vi "HFRR ADV v08 new software.vi"() -> ()   [LabVIEW 2025] (continued)
          n1265 = Read from Text File "Read File"(file (use dialog)=w1584) -> (text=w1583:string)  [unwired: 3 in, 3 out]
          n1266 = Match Pattern(string=w1583, regular expression="]") -> (after substring=w1581:string)  [unwired: 1 in, 3 out]
          n1267 = String Subset(string=w1583, offset (0)=5, length (rest)=10 ("length (rest)")) -> (substring=w1576:string)
          n1268 = Fract/Exp String To Number(string=w1576) -> (number=w1577:dbl)  [unwired: 3 in, 1 out]
          n1269 = Match Pattern(string=w1581, regular expression="-") -> (before substring=w1579:string)  [unwired: 1 in, 3 out]
          n1270 = case shown="19" w1578 {
            tunnel: w1577 -> [w1587 w1588 w1589 w1590 _ _ _ w1595 w1596 _ w1597 w1598 w1599 w1600 w1601 w1602 _ w1603 w1604 _ _ _ _ _]
            tunnel: w1579 -> [_ _ _ _ w1591 w1592 w1593 _ _ _ _ _ _ _ _ _ _ _ _ w1605 w1606 w1607 w1608 _]
            frame 0 {
              n1271 = local write "FRIC. FORCE :"(w1587) -> ()
            }
            frame 1 {
              n1272 = local write "TEMPERATURE :"(w1588) -> ()
            }
            frame 2 {
              n1273 = local write "HUMIDITY:"(w1589) -> ()
            }
            frame 3 {
              n1274 = local write "AIR TEMPERATURE :"(w1590) -> ()
            }
            frame 4 {
              n1275 = local write "Com Port 1"(w1591) -> ()
            }
            frame 5 {
              n1276 = local write "Com Port 2"(w1592) -> ()
              n1277 = local write "visa due"(w1592) -> ()
            }
            frame 6 {
              n1278 = String To Path(string=w1593) -> (path=w1594:path)
              n1279 = local write "File Path"(w1594) -> ()
              "String" <- w1593
            }
            frame 7 {
              n1280 = local write "DISPLACEMENT :"(w1595) -> ()
            }
            frame 8 {
              n1281 = local write "STROKE GAIN :"(w1596) -> ()
            }
            frame 9 {
            }
            frame 10 {
              n1282 = local write "Language Selection"(w1597) -> ()
            }
            frame 11 {
              n1283 = local write "CH-POWER +"(w1598) -> ()
            }
            frame 12 {
              n1284 = local write "CH-POWER -"(w1599) -> ()
            }
            frame 13 {
              n1285 = local write "CH-HEATER"(w1600) -> ()
            }
            frame 14 {
              n1286 = local write "CH-HUMIDITY WET"(w1601) -> ()
            }
            frame 15 {
              n1287 = local write "CH-HUMIDITY DRY"(w1602) -> ()
            }
            frame 16 {
            }
            frame 17 {
              n1288 = local write "AIR TEMP INTERCEPT:"(w1603) -> ()
            }
            frame 18 {
              n1289 = local write "TEMP INTERCEPT:"(w1604) -> ()
            }
            frame 21 {
              n1290 = local write "S.NO"(w1605) -> ()
            }
            frame 22 {
              n1291 = local write "Com Port 3"(w1606) -> ()
            }
            frame 20 {
              n1292 = local write "Camera Port :"(w1607) -> ()
            }
            frame 19 {
              n1293 = local write "C3 :"(w1608) -> ()
            }
            frame 23, Default {
            }
          }
        }
      }
    }
    n1294 = Select(t=u32 2500 ("milliseconds to wait"), s=w1561, f=u32 500 ("milliseconds to wait")) -> (s? t:f=w1559:u32)
    n1295 = Multiply(x=w1564, y=w1559) -> (x*y=w1566:dbl)
    n1296 = property on="Time slide" class="Slide (strict)"("Visible"=w1555) -> ()  [unwired: 2 in, 2 out]
    n1297 = call "Elapsed Time2"("Time Target (s)"=w1566, "Auto Reset"=TRUE) -> ("Time has Elapsed"=w1556:bool)  [unwired: 10 in, 7 out]
    n1298 = case shown="True" w1556 {
      frame False {
      }
      frame True {
        n1299 = stacked-sequence {
          frame #0 {
            # "DATA PROCESSING"
            # "115 mV/N"
            n1300 = local read "Sample Temperature"() -> (w1609:dbl)
            "TEMP 2" <- w1609
            "TEMP 3" <- w1609
            n1301 = local read "RH Numeric:"() -> (w1616:dbl)
            n1302 = local read "HUMIDITY:"() -> (w1617:dbl)
            n1303 = local read "FRICVALZ"() -> (w1628:dbl)
            n1304 = local read "Friction"() -> (w1612:dbl)
            n1305 = local write "TEMP"(w1609) -> ()
            n1306 = Multiply(x=w1616, y=w1617) -> (x*y=→"Humidity ( %RH )" →"Hum" →"Hum 2":dbl)
            n1307 = Subtract(x=w1612, y=w1628) -> (x-y=w1623:dbl)
            "FF 2" <- w1623
            "FF 4" <- w1623
            n1308 = local read "Ambient Temperature"() -> (→"AIR TEMP":dbl)
            n1309 = local read "TEMP"() -> (w1627:dbl)
            n1310 = local write "FF 3"(w1623) -> ()
            n1311 = Compound Arithmetic op=OR("FRICVALZ 4", "FRICVALZ 3", "FRICVALZ 2") -> (w1619:bool)
            n1312 = case shown="True" w1619 {
              tunnel: w1612 -> [_ w1634]
              frame False {
              }
              frame True {
                w1633 = FALSE ("FRICVALZ")
                n1313 = local write "FRICVALZ 3"(w1633) -> ()
                n1314 = local write "FRICVALZ 2"(w1633) -> ()
                n1315 = local write "FRICVALZ 4"(w1633) -> ()
                "FRICVALZ" <- w1634
              }
            }
            n1316 = Not A Number/Path/Refnum?(number/path/refnum=w1627) -> (NaN/Path/Refnum?=w1626:bool)
            n1317 = Not A Number/Path/Refnum?(number/path/refnum=w1623) -> (NaN/Path/Refnum?=w1625:bool)
            n1318 = Divide(x=w1623, y=1.96) -> (x/y=w1620:dbl)
            n1319 = Compound Arithmetic op=OR(w1626, w1625) -> (w1624:bool)
            n1320 = Not A Number/Path/Refnum?(number/path/refnum=w1620) -> (NaN/Path/Refnum?=w1621:bool)
            n1321 = case shown="True" w1624 {
              frame False {
              }
              frame True {
                n1322 = local write "TEMP"(0.0 ("TEMP")) -> ()
                n1323 = local write "FF 2"(0.0 ("FF 2")) -> ()
                n1324 = local write "reinit"(TRUE ("reinit")) -> ()
              }
            }
            n1325 = Select(t=0.0, s=w1621, f=w1620) -> (s? t:f=w1611:dbl)
            "COF 2" <- w1611
            n1326 = local write "COF 3"(w1611) -> ()
          }
        }
      }
    }
    n1327 = Wait (ms)(milliseconds to wait=u32 50) -> ()  [unwired: 1 out]
    n1328 = local read "Quit"() -> (w1548:bool)
    "Rate" <- 2500.0 ("No of Samples")
  }
  n1329 = while {
    tunnel: w57 -> [_]
    tunnel: [w1661] -> _
    tunnel: [w1637] -> w56
    i -> [w1661]
    stop <- w1637 stop-if-true
    # "C:\\LAB-IQ-NXT\\Scar View.exe"
    n1330 = local read "OK Button 16"() -> (w1650:bool)
    n1331 = local read "Main Tab"() -> (w1643:T2)
    n1332 = local read "service 3"() -> (w1644:bool)
    n1333 = local read "OPEN 6"() -> (w1646:bool)
    n1334 = local read "EDIT 2"() -> (w1648:bool)
    n1335 = flat-sequence {
      frame #0 {
        n1336 = local read "SAVE 2"() -> (w2263:bool)
        n1337 = stacked-sequence {
          frame #0 {
            n1338 = local read "EDIT"() -> (w2317:bool)
            n1339 = case shown="True" w2317 {
              tunnel: [u8 2 ("Disabled") u8 0 ("Disabled")] -> _
              frame False {
                w2319 = FALSE
                n1340 = local write "Password"("") -> ()
                n1341 = property on="SrvM CP" class="Bool (strict)"("Visible"=w2319) -> ()  [unwired: 2 in, 2 out]
                n1342 = property on="message" class="Str"("Visible"=w2319) -> ()  [unwired: 2 in, 2 out]
                n1343 = local write "x = y?"(w2319) -> ()
                n1344 = property on="Password" class="Str"("Visible"=w2319) -> ()  [unwired: 2 in, 2 out]
                n1345 = property on="ENTER THE NEW PASSWORD" class="Str"("Visible"=w2319) -> ()  [unwired: 2 in, 2 out]
                n1346 = property on="ENTER CURRENT PASSWORD" class="Str"("Visible"=w2319) -> ()  [unwired: 2 in, 2 out]
                n1347 = local write "SrvM CP"(w2319) -> ()
              }
              frame True {
                w2322 = TRUE
                n1348 = property on="SrvM CP" class="Bool (strict)"("Visible"=w2322) -> ()  [unwired: 2 in, 2 out]
                n1349 = property on="Password" class="Str"("Visible"=w2322) -> ()  [unwired: 2 in, 2 out]
              }
            }
            "dipl pwd" <- "@143$\n" ("dipl pwd")
          }
          frame #1 {
            # "Gain password"
            n1350 = String To Byte Array(string="ENTER CURRENT PASSWORD") -> (unsigned byte array=w2327:u8[])
            n1351 = Search 1D Array(1D array=w2327, element=u8 10) -> (index of element=w2330:i32)  [unwired: 1 in]
            n1352 = Index Array(array=w2327, index=w2330) -> (element=w2326:u8)
            n1353 = Equal?(x=w2326, y=10) -> (x = y?=w2324:bool)
            n1354 = case shown="True" w2324 {
              frame False {
                n1355 = property on="ENTER THE NEW PASSWORD" class="Str"("Visible"=FALSE) -> ()  [unwired: 2 in, 2 out]
              }
              frame True {
                # "password"
                # "change password logic"
                n1356 = local read "ENTER CURRENT PASSWORD"() -> (w2343:string)
                n1357 = local read "dipl pwd"() -> (w2337:string)
                n1358 = String To Byte Array(string=w2343) -> (unsigned byte array=w2345:u8[])
                n1359 = String To Byte Array(string=w2337) -> (unsigned byte array=w2338:u8[])
                n1360 = Array Size(array=w2345) -> (size(s)=w2342:i32)
                n1361 = Array Size(array=w2338) -> (size(s)=w2340:i32)
                n1362 = for {
                  N: w2342 -> [_]
                  tunnel: w2345 -> [w2369]
                  tunnel: [w2367] -> w2346 mode=indexing
                  tunnel: w2342 -> [w2361]
                  i -> [w2362]
                  n1363 = Decrement(x=w2361) -> (x-1=w2359:i32)
                  n1364 = Equal?(x=w2362, y=w2359) -> (x = y?=w2360:bool)
                  n1365 = Index Array(array=w2369, index=w2362) -> (element=w2363:u8)
                  n1366 = Number To Decimal String(number=w2363) -> (decimal integer string=w2368:string)  [unwired: 1 in]
                  n1367 = Select(t="", s=w2360, f="\r") -> (s? t:f=w2365:string)
                  n1368 = Concatenate Strings(w2368, w2365) -> (w2367:string)
                }
                n1369 = for {
                  N: w2340 -> [_]
                  tunnel: w2338 -> [w2357]
                  tunnel: [w2355] -> w2339 mode=indexing
                  tunnel: w2340 -> [w2352]
                  i -> [w2353]
                  n1370 = Decrement(x=w2352) -> (x-1=w2351:i32)
                  n1371 = Equal?(x=w2353, y=w2351) -> (x = y?=w2350:bool)
                  n1372 = Index Array(array=w2357, index=w2353) -> (element=w2356:u8)
                  n1373 = Number To Decimal String(number=w2356) -> (decimal integer string=w2354:string)  [unwired: 1 in]
                  n1374 = Select(t="", s=w2350, f="\r") -> (s? t:f=w2347:string)
                  n1375 = Concatenate Strings(w2354, w2347) -> (w2355:string)
                }
                n1376 = local read "string"() -> (w2344:string)
                n1377 = Concatenate Strings(w2339) -> (w2333:string)
                n1378 = Concatenate Strings(w2344) -> (w2341:string)
                n1379 = Concatenate Strings(w2346) -> (w2334:string)
                n1380 = Equal?(x=w2334, y=w2341) -> (x = y?=w2336:bool)
                n1381 = Equal?(x=w2334, y=w2333) -> (x = y?=w2332:bool)
                n1382 = Or(x=w2336, y=w2332) -> (x .or. y?=w2335:bool)
                n1383 = case shown="True" w2335 {
                  frame False {
                  }
                  frame True {
                    n1384 = property on="ENTER THE NEW PASSWORD" class="Str"("Visible"=TRUE) -> ()  [unwired: 2 in, 2 out]
                  }
                }
              }
            }
          }
          frame #2 {
            n1385 = String To Byte Array(string="ENTER THE NEW PASSWORD") -> (unsigned byte array=w2372:u8[])
            n1386 = Search 1D Array(1D array=w2372, element=u8 10) -> (index of element=w2376:i32)  [unwired: 1 in]
            n1387 = Index Array(array=w2372, index=w2376) -> (element=w2374:u8)
            n1388 = Equal?(x=w2374, y=10) -> (x = y?=w2371:bool)
            n1389 = case shown="False" w2371 {
              frame False {
              }
              frame True {
                n1390 = local write "EDIT"(FALSE) -> ()
                n1391 = local write "SrvM CP"(FALSE) -> ()
                n1392 = local read "ENTER THE NEW PASSWORD"() -> (w2379:string)
                n1393 = String To Byte Array(string=w2379) -> (unsigned byte array=w2384:u8[])
                n1394 = Array Size(array=w2384) -> (size(s)=w2381:i32)
                n1395 = for {
                  N: w2381 -> [_]
                  tunnel: w2384 -> [w2397]
                  tunnel: [w2394] -> w2386 mode=indexing
                  tunnel: w2381 -> [w2389]
                  i -> [w2387]
                  n1396 = Decrement(x=w2389) -> (x-1=w2390:i32)
                  n1397 = Equal?(x=w2387, y=w2390) -> (x = y?=w2391:bool)
                  n1398 = Index Array(array=w2397, index=w2387) -> (element=w2396:u8)
                  n1399 = Number To Decimal String(number=w2396) -> (decimal integer string=w2395:string)  [unwired: 1 in]
                  n1400 = Select(t="", s=w2391, f="\r") -> (s? t:f=w2388:string)
                  n1401 = Concatenate Strings(w2395, w2388) -> (w2394:string)
                }
                n1402 = local read "file path"() -> (w2378:path)
                n1403 = Concatenate Strings(w2386) -> (w2380:string)
                n1404 = Delete(path (use dialog)=w2378) -> (deleted path=w2382:path)  [unwired: 4 in, 2 out]
                n1405 = call <vilib>:"Write Characters To File.vi"("append to file? (new file:F)"=FALSE, "character string"=w2380, "file path (dialog if empty)"=w2382) -> ()  [unwired: 2 in, 1 out]
              }
            }
          }
          frame #3 {
            n1406 = case shown="True" "SrvM CP" {
              frame False {
                w2400 = ""
                n1407 = local write "ENTER CURRENT PASSWORD"(w2400) -> ()
                n1408 = local write "ENTER THE NEW PASSWORD"(w2400) -> ()
                n1409 = property on="ENTER CURRENT PASSWORD" class="Str"("Visible"=FALSE) -> ()  [unwired: 2 in, 2 out]
              }
              frame True {
                n1410 = property on="ENTER THE NEW PASSWORD" class="Str"() -> ("Visible"=w2401:bool)  [unwired: 2 in, 2 out]
                n1411 = Not(x=w2401) -> (.not. x?=w2402:bool)
                n1412 = property on="ENTER CURRENT PASSWORD" class="Str"("Visible"=w2402) -> ()  [unwired: 2 in, 2 out]
              }
            }
          }
          frame #4 {
            n1413 = String To Byte Array(string="Password") -> (unsigned byte array=w2409:u8[])
            n1414 = Search 1D Array(1D array=w2409, element=u8 10) -> (index of element=w2407:i32)  [unwired: 1 in]
            n1415 = Index Array(array=w2409, index=w2407) -> (element=w2408:u8)
            n1416 = Equal?(x=w2408, y=10) -> (x = y?=w2404:bool)
            n1417 = case shown="True" w2404 {
              frame False {
              }
              frame True {
                # "password"
                # "password"
                n1418 = local read "Password"() -> (w2422:string)
                n1419 = String To Byte Array(string=w2422) -> (unsigned byte array=w2425:u8[])
                n1420 = String To Byte Array(string="@143$\n") -> (unsigned byte array=w2411:u8[])
                n1421 = Array Size(array=w2425) -> (size(s)=w2420:i32)
                n1422 = Array Size(array=w2411) -> (size(s)=w2416:i32)
                n1423 = for {
                  N: w2420 -> [_]
                  tunnel: w2425 -> [w2459]
                  tunnel: [w2457] -> w2426 mode=indexing
                  tunnel: w2420 -> [w2454]
                  i -> [w2455]
                  n1424 = Decrement(x=w2454) -> (x-1=w2453:i32)
                  n1425 = Index Array(array=w2459, index=w2455) -> (element=w2458:u8)
                  n1426 = Equal?(x=w2455, y=w2453) -> (x = y?=w2452:bool)
                  n1427 = Number To Decimal String(number=w2458) -> (decimal integer string=w2456:string)  [unwired: 1 in]
                  n1428 = Select(t="", s=w2452, f="\r") -> (s? t:f=w2449:string)
                  n1429 = Concatenate Strings(w2456, w2449) -> (w2457:string)
                }
                n1430 = for {
                  N: w2416 -> [_]
                  tunnel: w2411 -> [w2470]
                  tunnel: [w2468] -> w2414 mode=indexing
                  tunnel: w2416 -> [w2465]
                  i -> [w2466]
                  n1431 = Decrement(x=w2465) -> (x-1=w2464:i32)
                  n1432 = Index Array(array=w2470, index=w2466) -> (element=w2469:u8)
                  n1433 = Equal?(x=w2466, y=w2464) -> (x = y?=w2463:bool)
                  n1434 = Number To Decimal String(number=w2469) -> (decimal integer string=w2467:string)  [unwired: 1 in]
                  n1435 = Select(t="", s=w2463, f="\r") -> (s? t:f=w2460:string)
                  n1436 = Concatenate Strings(w2467, w2460) -> (w2468:string)
                }
                n1437 = local read "file path"() -> (w2410:path)
                n1438 = call <vilib>:"Read Characters From File.vi"("file path (dialog if empty)"=w2410) -> ("character string"=w2424:string)  [unwired: 5 in, 3 out]
                "string" <- w2424
                n1439 = flat-sequence {
                  tunnel: [w2427] -> w2421
                  frame #0 {
                    w2427 = ""
                    n1440 = local write "Password"(w2427) -> ()
                  }
                }
                n1441 = Concatenate Strings(w2414) -> (w2415:string)
                n1442 = Concatenate Strings(w2424) -> (w2423:string)
                n1443 = Concatenate Strings(w2426) -> (w2418:string)
                n1444 = Equal?(x=w2418, y=w2423) -> (x = y?=w2413:bool)
                n1445 = Equal?(x=w2418, y=w2415) -> (x = y?=w2419:bool)
                n1446 = Or(x=w2413, y=w2419) -> (x .or. y?=w2412:bool)
                "x = y?" <- w2412
                n1447 = case shown="True" w2412 {
                  selector: w2412 -> [w2429 _]
                  tunnel: w2421 -> [_ _]
                  frame False {
                    n1448 = And(x=w2429, y=TRUE ("Visible")) -> (x .and. y?=w2430:bool)
                    n1449 = property on="message" class="Str"("Visible"=w2430) -> ()  [unwired: 2 in, 2 out]
                  }
                  frame True {
                    n1450 = control-ref of="This VI"() -> (w2441:refnum<vi>)
                    n1451 = property class="VI"(reference=w2441) -> (reference out=w2432:refnum<vi>, error out=w2436:errorcluster, "Panel"=w2440:refnum<vi>)  [unwired: 1 in]
                    n1452 = property on="message" class="Str"("Visible"=FALSE) -> ()  [unwired: 2 in, 2 out]
                    n1453 = property class="Pnl"(reference=w2440, error in=w2436) -> (reference out=w2434:refnum<vi>, error out=w2437:errorcluster, "Panes[]"=w2439:refnum<vi>[])
                    n1454 = for {
                      tunnel: w2439 -> [w2448] mode=indexing
                      tunnel: T19."Always On" ("Horizontal Scrollbar Visibility") -> [w2447]
                      tunnel: w2437 -> [w2444]
                      tunnel: [w2443] -> w2435
                      n1455 = property class="Pane"(reference=w2448, error in=w2444, "HorizScrollbarVisibility"=w2447) -> (reference out=w2445:refnum<vi>, error out=w2446:errorcluster)
                      n1456 = Close Reference(reference=w2445, error in (no error)=w2446) -> (error out=w2443:errorcluster)
                    }
                    n1457 = Close Reference(reference=w2434, error in (no error)=w2435) -> (error out=w2433:errorcluster)
                    n1458 = Close Reference(reference=w2432, error in (no error)=w2433) -> (error out=→"error out 6":errorcluster)
                  }
                }
              }
            }
          }
        }
        n1459 = local read "x = y?"() -> (w2269:bool)
        n1460 = local read "HUMIDITY: 2"() -> (w2271:dbl)
        n1461 = local read "HUMIDITY:"() -> (w2270:dbl)
        n1462 = property on="Port 2 Error" class="Clust (strict)"("Visible"="EDIT") -> ()  [unwired: 2 in, 2 out]
        n1463 = property on="Port 1 Error" class="Clust (strict)"("Visible"="EDIT") -> ()  [unwired: 2 in, 2 out]
        n1464 = case shown="True" "SrvM CP 2" {
          frame False {
          }
          frame True {
            n1465 = local write "SrvM CP 2"(FALSE ("SrvM CP 2")) -> ()
            n1466 = local read "HUMIDITY: 2"() -> (w2310:dbl)
            n1467 = local read "TEMP INTERCEPT: 2"() -> (w2309:dbl)
            n1468 = local read "DISPLACEMENT : 4"() -> (w2313:dbl)
            n1469 = local read "TEMPERATURE : 2"() -> (w2312:dbl)
            n1470 = local read "STROKE GAIN : 2"() -> (w2314:dbl)
            n1471 = local read "FRIC. FORCE : 2"() -> (w2315:dbl)
            n1472 = local read "AIR TEMP INTERCEPT: 2"() -> (w2308:dbl)
            n1473 = local read "AIR TEMPERATURE : 2"() -> (w2311:dbl)
            n1474 = local write "HUMIDITY:"(w2310) -> ()
            n1475 = local write "AIR TEMP INTERCEPT:"(w2309) -> ()
            n1476 = local write "TEMPERATURE :"(w2312) -> ()
            n1477 = local write "FRIC. FORCE :"(w2315) -> ()
            n1478 = local write "STROKE GAIN :"(w2314) -> ()
            n1479 = local write "DISPLACEMENT :"(w2313) -> ()
            n1480 = local write "AIR TEMPERATURE :"(w2311) -> ()
            n1481 = local write "TEMP INTERCEPT:"(w2308) -> ()
          }
        }
        n1482 = Or(x="SAVE", y=w2263) -> (x .or. y?=w2264:bool)
        n1483 = And(x="EDIT", y=w2269) -> (x .and. y?=w2267:bool)
        n1484 = local read "DISPLACEMENT : 4"() -> (w2280:dbl)
        n1485 = local read "TEMPERATURE : 2"() -> (w2278:dbl)
        n1486 = local read "STROKE GAIN : 2"() -> (w2284:dbl)
        n1487 = local read "DISPLACEMENT :"() -> (w2279:dbl)
        n1488 = local read "FRIC. FORCE : 2"() -> (w2287:dbl)
        n1489 = local read "TEMPERATURE :"() -> (w2276:dbl)
        n1490 = local read "STROKE GAIN :"() -> (w2283:dbl)
        n1491 = local read "FRIC. FORCE :"() -> (w2286:dbl)
        n1492 = case shown="True" w2267 {
          tunnel: [u8 2 ("Disabled") u8 0 ("Disabled")] -> w2266
          tunnel: [w2631 TRUE ("Visible")] -> w2265
          frame False {
            w2631 = FALSE ("Visible")
            n1493 = local write "EDIT 2"(w2631) -> ()
          }
          frame True {
          }
        }
        n1494 = case shown="True" w2264 {
          frame False {
          }
          frame True {
            n1495 = stacked-sequence {
              seq-local: [w2479 _ _] -> [_ w2626 _]
              frame #0 {
                (unwired) i16 5 ("precision (6)")
                # "[CH1]    - FF\n[CH2]   - TEMPERATURE\n[CH3]    - Humidity\n[CH4]    - AIR TEMP\n[CH5]\\- Visa Uno\n[CH6] \\- Visa Due\n[CH7]  \\- file path\n[CH8]   - Displacement Gain\n[CHA]   - Stroke Gain\n[CHB]   - Stroke PID Gain\n[CHC]   -Language Selection\n[CHD]   -Power +\n[CHE]   -Power_\n[CHF]   -Heater\n[CHG]   -Humidity Wet\n[CHH]   -Humidity Dry\n[CHI]   -Integral Time"
                n1496 = local read "Language Selection"() -> (w2527:enum16{"English", "Russian"})
                n1497 = local read "CH-HUMIDITY WET"() -> (w2485:u16)
                n1498 = local read "CH-HUMIDITY DRY"() -> (w2482:u16)
                n1499 = local read "STROKE GAIN :"() -> (w2471:dbl)
                n1500 = local read "CH-POWER +"() -> (w2494:u16)
                n1501 = local read "CH-POWER -"() -> (w2491:u16)
                n1502 = local read "CH-HEATER"() -> (w2488:u16)
                n1503 = local read "AIR TEMPERATURE :"() -> (w2474:dbl)
                n1504 = local read "DISPLACEMENT :"() -> (w2472:dbl)
                n1505 = local read "TEMPERATURE :"() -> (w2475:dbl)
                n1506 = local read "FRIC. FORCE :"() -> (w2476:dbl)
                n1507 = local read "HUMIDITY:"() -> (w2473:dbl)
                n1508 = Path To String(path="File Path") -> (string=w2543:string)
                n1509 = Number To Fractional String(number=w2471, width (-)=i16 10 ("precision (6)"), precision (6)=i16 5) -> (F-format string=w2534:string)  [unwired: 1 in]
                n1510 = Number To Fractional String(number=w2527, width (-)=i16 10 ("precision (6)"), precision (6)=i16 5) -> (F-format string=w2523:string)  [unwired: 1 in]
                n1511 = Number To Fractional String(number=w2494, width (-)=i16 10 ("precision (6)"), precision (6)=i16 5) -> (F-format string=w2517:string)  [unwired: 1 in]
                n1512 = Number To Fractional String(number=w2491, width (-)=i16 10 ("precision (6)"), precision (6)=i16 5) -> (F-format string=w2514:string)  [unwired: 1 in]
                n1513 = Number To Fractional String(number=w2488, width (-)=i16 10 ("precision (6)"), precision (6)=i16 5) -> (F-format string=w2509:string)  [unwired: 1 in]
                n1514 = Number To Fractional String(number=w2485, width (-)=i16 10 ("precision (6)"), precision (6)=i16 5) -> (F-format string=w2506:string)  [unwired: 1 in]
                n1515 = Number To Fractional String(number=w2482, width (-)=i16 10 ("precision (6)"), precision (6)=i16 5) -> (F-format string=w2501:string)  [unwired: 1 in]
                n1516 = local read "Com Port 1"() -> (w2478:refnum<visa-resource-name>)
                n1517 = local read "Com Port 2"() -> (w2477:refnum<visa-resource-name>)
                n1518 = Concatenate Strings(w2543, "\\" ("string")) -> (w2542:string)
                n1519 = Number To Fractional String(number=w2476, width (-)=i16 10 ("precision (6)"), precision (6)=i16 5) -> (F-format string=w2575:string)  [unwired: 1 in]
                n1520 = Number To Fractional String(number=w2475, width (-)=i16 10 ("precision (6)"), precision (6)=i16 5) -> (F-format string=w2574:string)  [unwired: 1 in]
                n1521 = Number To Fractional String(number=w2473, width (-)=i16 10 ("precision (6)"), precision (6)=i16 5) -> (F-format string=w2568:string)  [unwired: 1 in]
                n1522 = Number To Fractional String(number=w2474, width (-)=i16 10 ("precision (6)"), precision (6)=i16 5) -> (F-format string=w2562:string)  [unwired: 1 in]
                n1523 = Number To Fractional String(number=w2472, width (-)=i16 10 ("precision (6)"), precision (6)=i16 5) -> (F-format string=w2535:string)  [unwired: 1 in]
                n1524 = Concatenate Strings("[CHA]" ("string"), w2534, "- Stroke Gain" ("string"), "\r") -> (w2528:string)
                n1525 = Concatenate Strings("[CHC]" ("string"), w2523, "-Language Selection" ("string"), "\r") -> (w2520:string)
                n1526 = Concatenate Strings("[CHD]" ("string"), w2517, "-Power +" ("string"), "\r") -> (w2499:string)
                n1527 = Concatenate Strings("[CHG]" ("string"), w2506, "-Humidity Wet" ("string"), "\r") -> (w2496:string)
                n1528 = Concatenate Strings("[CHH]" ("string"), w2501, "-Humidity Dry" ("string"), "\r") -> (w2495:string)
                n1529 = Concatenate Strings("[CH1]" ("string"), w2575, " - FF" ("string"), "\r") -> (w2573:string)
                n1530 = Concatenate Strings("[CH2]" ("string"), w2574, " - TEMPERATURE" ("string"), "\r") -> (w2572:string)
                n1531 = Concatenate Strings("[CH3]" ("string"), w2568, " - Humidity" ("string"), "\r") -> (w2565:string)
                n1532 = Concatenate Strings("[CH4]" ("string"), w2562, " - AIR TEMP" ("string"), "\r") -> (w2558:string)
                n1533 = Concatenate Strings("[CH5]" ("string"), w2478, "- Visa Uno" ("string"), "\r") -> (w2551:string)
                n1534 = Concatenate Strings("[CH6]" ("string"), w2477, "- Visa Due" ("string"), "\r") -> (w2546:string)
                n1535 = Concatenate Strings("[CH7]" ("string"), w2542, "- file path" ("string"), "\r") -> (w2545:string)
                n1536 = Concatenate Strings("[CH8]" ("string"), w2535, "- Displacement Gain" ("string"), "\r") -> (w2538:string)
                n1537 = Concatenate Strings("[CHE]" ("string"), w2514, "-Power_" ("string"), "\r") -> (w2498:string)
                n1538 = Concatenate Strings("[CHF]" ("string"), w2509, "-Heater" ("string"), "\r") -> (w2497:string)
                n1539 = Concatenate Strings(w2573, w2572, w2565, w2558, w2551, w2546, w2545, w2538, w2528, w2520, w2499, w2498, w2497, w2496, w2495) -> (w2479:string)
                "gain" <- w2479
              }
              frame #1 {
                n1540 = local read "Camera Port :"() -> (w2587:string)
                n1541 = local read "C3 :"() -> (w2595:refnum<visa-resource-name>)
                n1542 = local read "TEMP INTERCEPT:"() -> (w2596:dbl)
                n1543 = local read "AIR TEMP INTERCEPT:"() -> (w2597:dbl)
                n1544 = local read "Com Port 3"() -> (w2598:refnum<visa-resource-name>)
                n1545 = Concatenate Strings("[CH8]" ("string"), w2587, "- Visa Camera" ("string"), "\r") -> (w2586:string)
                n1546 = Concatenate Strings("[CH7]" ("string"), w2595, "- Visa Humidity" ("string"), "\r") -> (w2591:string)
                n1547 = Number To Fractional String(number=w2596, width (-)=i16 10 ("precision (6)"), precision (6)=i16 5) -> (F-format string=w2614:string)  [unwired: 1 in]
                n1548 = Concatenate Strings("[CHL]" ("string"), w2598, "- Visa humid" ("string"), "\r") -> (w2601:string)
                n1549 = Number To Fractional String(number=w2597, width (-)=i16 10 ("precision (6)"), precision (6)=i16 5) -> (F-format string=w2621:string)  [unwired: 1 in]
                n1550 = Concatenate Strings("[CHK]" ("string"), w2614, "-TEMP INTERCEPT" ("string"), "\r") -> (w2610:string)
                n1551 = Concatenate Strings("[SNO]" ("string"), "S.NO", "-" ("string"), "\r") -> (w2606:string)
                n1552 = Concatenate Strings("[CHJ]" ("string"), w2621, "-AIR TEMP INTERCEPT" ("string"), "\r") -> (w2611:string)
                n1553 = String To Path(string="C:\\LAB-IQ\\calibrate WO 2465.dcf") -> (path=w2599:path)
                n1554 = Concatenate Strings(w2626, w2611, w2610, w2606, w2601, w2591, w2586) -> (w2625:string)
                n1555 = call <vilib>:"Write Characters To File.vi"("append to file? (new file:F)"=FALSE, "character string"=w2625, "file path (dialog if empty)"=w2599) -> ()  [unwired: 2 in, 1 out]
              }
              frame #2 {
                n1556 = local write "Lan flag"(0.0 ("Lan flag")) -> ()
                n1557 = local write "conststatus"(0.0 ("rpm value : 2")) -> ()
                n1558 = local write "SAVE"(FALSE ("OK Button 14")) -> ()
                n1559 = local write "SAVE 2"(FALSE ("SAVE 2")) -> ()
              }
            }
          }
        }
        n1560 = Subtract(x=w2271, y=w2270) -> (x-y=w2272:dbl)
        n1561 = local read "AIR TEMPERATURE : 2"() -> (w2275:dbl)
        n1562 = local read "AIR TEMPERATURE :"() -> (w2274:dbl)
        n1563 = Divide(x=w2272, y=w2270) -> (x/y=w2294:dbl)
        n1564 = Subtract(x=w2287, y=w2286) -> (x-y=w2285:dbl)
        n1565 = Subtract(x=w2278, y=w2276) -> (x-y=w2277:dbl)
        n1566 = Subtract(x=w2284, y=w2283) -> (x-y=w2282:dbl)
        n1567 = Subtract(x=w2280, y=w2279) -> (x-y=w2281:dbl)
        n1568 = Subtract(x=w2275, y=w2274) -> (x-y=w2273:dbl)
        n1569 = Divide(x=w2285, y=w2286) -> (x/y=w2305:dbl)
        n1570 = Divide(x=w2277, y=w2276) -> (x/y=w2298:dbl)
        n1571 = Divide(x=w2282, y=w2283) -> (x/y=w2302:dbl)
        n1572 = Divide(x=w2281, y=w2279) -> (x/y=w2301:dbl)
        n1573 = Multiply(x=w2294, y=100.0) -> (x*y=→"HUMIDITY  Calibration Error":dbl)
        n1574 = Divide(x=w2273, y=w2274) -> (x/y=w2297:dbl)
        n1575 = Multiply(x=w2305, y=100.0) -> (x*y=→"FRIC. FORCE Calibration Error":dbl)
        n1576 = Multiply(x=w2298, y=100.0) -> (x*y=→"TEMPERATURE  Calibration Error":dbl)
        n1577 = Multiply(x=w2302, y=100.0) -> (x*y=→"STROKE Calibration Error":dbl)
        n1578 = Multiply(x=w2301, y=100.0) -> (x*y=→"DISPLACEMENT  Calibration Error":dbl)
        n1579 = property on="EDIT 2" class="Bool (strict)"("Visible"=w2265) -> ()  [unwired: 2 in, 2 out]
        n1580 = property on="SAVE" class="Bool (strict)"("Visible"=w2265) -> ()  [unwired: 2 in, 2 out]
        n1581 = property on="SrvM CP" class="Bool (strict)"("Disabled"=w2266) -> ()  [unwired: 2 in, 2 out]
        n1582 = property on="visa due" class="CmbBox"("Disabled"=w2266) -> ()  [unwired: 2 in, 2 out]
        n1583 = property on="File Path" class="Path"("Disabled"=w2266) -> ()  [unwired: 2 in, 2 out]
        n1584 = Multiply(x=w2297, y=100.0) -> (x*y=→"AIR TEMPERATURE  Calibration Error":dbl)
        n1585 = property on="Language Selection" class="Enum (strict)"("Visible"=w2265) -> ()  [unwired: 2 in, 2 out]
        n1586 = property on="Tab Control 7" class="TabCtl (strict)"("Disabled"=w2266) -> ()  [unwired: 2 in, 2 out]
        n1587 = property on="AIR TEMP INTERCEPT:" class="DigNum (strict)"("Disabled"=w2266) -> ()  [unwired: 2 in, 2 out]
        n1588 = property on="CH-POWER -" class="DigNum (strict)"("Disabled"=w2266) -> ()  [unwired: 2 in, 2 out]
        n1589 = property on="CH-POWER +" class="DigNum (strict)"("Disabled"=w2266) -> ()  [unwired: 2 in, 2 out]
        n1590 = property on="AIR TEMPERATURE :" class="DigNum (strict)"("Disabled"=w2266) -> ()  [unwired: 2 in, 2 out]
        n1591 = property on="STROKE GAIN :" class="DigNum (strict)"("Disabled"=w2266) -> ()  [unwired: 2 in, 2 out]
        n1592 = property on="SPEED OUT:" class="DigNum (strict)"("Disabled"=w2266) -> ()  [unwired: 2 in, 2 out]
        n1593 = property on="CH-HUMIDITY DRY" class="DigNum (strict)"("Disabled"=w2266) -> ()  [unwired: 2 in, 2 out]
        n1594 = property on="HUMIDITY:" class="DigNum (strict)"("Disabled"=w2266) -> ()  [unwired: 2 in, 2 out]
        n1595 = property on="CH-HUMIDITY WET" class="DigNum (strict)"("Disabled"=w2266) -> ()  [unwired: 2 in, 2 out]
        n1596 = property on="TEMPERATURE :" class="DigNum (strict)"("Disabled"=w2266) -> ()  [unwired: 2 in, 2 out]
        n1597 = property on="DISPLACEMENT :" class="DigNum (strict)"("Disabled"=w2266) -> ()  [unwired: 2 in, 2 out]
        n1598 = property on="CH-HEATER" class="DigNum (strict)"("Disabled"=w2266) -> ()  [unwired: 2 in, 2 out]
        n1599 = property on="TEMP INTERCEPT:" class="DigNum (strict)"("Disabled"=w2266) -> ()  [unwired: 2 in, 2 out]
        n1600 = property on="FRIC. FORCE :" class="DigNum (strict)"("Disabled"=w2266) -> ()  [unwired: 2 in, 2 out]
      }
    }
    n1601 = local read "RUN"() -> (w1660:bool)
    n1602 = local read "RUN"() -> (w1658:bool)
    n1603 = disable-structure shown="Disabled" {
      disable-tunnel: [w1675 _] -> w1641
      disable-tunnel: [w1674 _] -> w1639
      frame Disabled {
        n1604 = local read "Temperature before test"() -> (w1668:dbl)
        n1605 = local read "Temperature after test"() -> (w1681:dbl)
        n1606 = case shown="True" "Save Results" {
          frame False {
          }
          frame True {
            w1697 = "\r"
            n1607 = local write "Save Results"(FALSE ("OK Button 5")) -> ()
            n1608 = local read "Temperature before test"() -> (w1735:dbl)
            n1609 = local read "Temperature after test"() -> (w1737:dbl)
            n1610 = local read "Humidity before test"() -> (w1734:dbl)
            n1611 = local read "Humidity after test"() -> (w1736:dbl)
            n1612 = local read "WS1.4"() -> (w1741:dbl)
            n1613 = local read "AVP"() -> (w1739:dbl)
            n1614 = Number To Fractional String(number=w1741, width (-)=i16 6, precision (6)=i16 1) -> (F-format string=w1701:string)  [unwired: 1 in]
            n1615 = local read "MWSD"() -> (w1738:dbl)
            n1616 = local read "String"() -> (w1730:string)
            n1617 = local read "FILE"() -> (w1733:string)
            n1618 = local read "HCF"() -> (w1740:dbl)
            n1619 = Number To Fractional String(number=w1734, width (-)=i16 6, precision (6)=i16 1) -> (F-format string=w1726:string)  [unwired: 1 in]
            n1620 = Number To Fractional String(number=w1735, width (-)=i16 6, precision (6)=i16 1) -> (F-format string=w1723:string)  [unwired: 1 in]
            n1621 = Number To Fractional String(number=w1736, width (-)=i16 6, precision (6)=i16 1) -> (F-format string=w1719:string)  [unwired: 1 in]
            n1622 = Number To Fractional String(number=w1737, width (-)=i16 6, precision (6)=i16 1) -> (F-format string=w1715:string)  [unwired: 1 in]
            n1623 = Number To Fractional String(number=w1739, width (-)=i16 6, precision (6)=i16 3) -> (F-format string=w1708:string)  [unwired: 1 in]
            n1624 = Concatenate Strings(w1730, w1733) -> (w1752:string)
            n1625 = Number To Fractional String(number=w1738, width (-)=i16 6, precision (6)=i16 1) -> (F-format string=w1712:string)  [unwired: 1 in]
            n1626 = Number To Fractional String(number=w1740, width (-)=i16 6, precision (6)=i16 2) -> (F-format string=w1706:string)  [unwired: 1 in]
            n1627 = Concatenate Strings("(" ("string"), w1701, ")Microns" ("string")) -> (w1700:string)
            n1628 = local read "REMARKS"() -> (w1732:string)
            "REMARKS 2" <- w1732
            n1629 = Concatenate Strings("(" ("string"), w1726, " ) % RH," ("string")) -> (w1727:string)
            n1630 = Concatenate Strings(w1706, ")" ("string")) -> (w1704:string)
            n1631 = Concatenate Strings("(" ("string"), w1723, ")  Deg C ," ("string")) -> (w1722:string)
            n1632 = Concatenate Strings("(" ("string"), w1719, " ) % RH," ("string")) -> (w1718:string)
            n1633 = Concatenate Strings("(" ("string"), w1715, ")  Deg C ," ("string")) -> (w1714:string)
            n1634 = Concatenate Strings("(" ("string"), w1712, ")  Microns," ("string")) -> (w1711:string)
            n1635 = Concatenate Strings("(" ("string"), w1708, ")  kPa," ("string")) -> (w1698:string)
            n1636 = Concatenate Strings(w1752, ".dwm" ("Substring")) -> (w1750:string)
            n1637 = String To Path(string=w1750) -> (path=w1749:path)
            n1638 = Concatenate Strings(w1732, w1697, " Humidity before test= " ("Substring"), w1727, w1697, " Temperature before test = " ("Substring"), w1722, w1697, " Humidity after test= " ("Substring"), w1718, w1697, "Temperature after test = " ("Substring"), w1714, w1697, "MSD = " ("Substring"), w1711, w1697, "  AVP = " ("Substring"), w1698, w1697, "  HCF                     =( " ("Substring"), w1704, w1697, " WS1.4                  = " ("Substring"), w1700, w1697) -> (w1696:string)
            "data" <- w1696
            n1639 = call <vilib>:"Write Characters To File.vi"("append to file? (new file:F)"=FALSE, "character string"=w1696, "file path (dialog if empty)"=w1749) -> ()  [unwired: 2 in, 1 out]
            n1640 = Match Pattern(string=w1696, regular expression="!") -> (after substring=→"export":string)  [unwired: 1 in, 3 out]
          }
        }
        n1641 = Add(x=231.864, y=w1668) -> (x+y=w1665:dbl)
        n1642 = Add(x=231.864, y=w1681) -> (x+y=w1678:dbl)
        n1643 = Divide(x=1705.984, y=w1665) -> (x/y=w1666:dbl)
        n1644 = Divide(x=1705.984, y=w1678) -> (x/y=w1679:dbl)
        n1645 = local read "Humidity before test"() -> (w1670:dbl)
        n1646 = local read "Humidity after test"() -> (w1683:dbl)
        n1647 = Subtract(x=8.017352 ("y"), y=w1666) -> (x-y=w1692:dbl)
        n1648 = Subtract(x=8.017352 ("y"), y=w1679) -> (x-y=w1686:dbl)
        n1649 = expression code="10**y"(w1692) -> (w1672:dbl)
        n1650 = expression code="10**y"(w1686) -> (w1685:dbl)
        n1651 = Multiply(x=w1670, y=w1672) -> (x*y=w1671:dbl)
        n1652 = Multiply(x=w1683, y=w1685) -> (x*y=w1684:dbl)
        n1653 = Divide(x=w1671, y=750.0) -> (x/y=w1687:dbl)
        n1654 = Divide(x=w1684, y=750.0) -> (x/y=w1688:dbl)
        n1655 = Add(x=w1687, y=w1688) -> (x+y=w1689:dbl)
        n1656 = Divide(x=w1689, y=2.0) -> (x/y=w1691:dbl)
        n1657 = local write "AVP"(w1691) -> ()
        n1658 = Subtract(x=1.4, y=w1691) -> (x-y=w1674:dbl)
        n1659 = local read "HCF"() -> (w1675:dbl)
      }
      frame Enabled {
      }
    }
    n1660 = case shown="True" "EDIT 3" {
      frame False {
      }
      frame True {
        n1661 = local write "EDIT 3"(FALSE ("EDIT 3")) -> ()
        n1662 = local write "Main Tab"(T2."About" ("Main Tab")) -> ()
      }
    }
    n1663 = case shown="False" w1660 {
      frame False {
        n1664 = local read "stopT"() -> (w2638:bool)
        n1665 = case shown="True" w2638 {
          frame False {
          }
          frame True {
            n1666 = local write "stopT"(FALSE) -> ()
          }
        }
      }
      frame True {
        "stopT" <- TRUE
      }
    }
    n1667 = case shown="False" w1658 {
      frame False {
      }
      frame True {
      }
    }
    n1668 = case shown="True" w1648 {
      frame False {
        n1669 = property on="Password 2" class="Str"("Visible"=FALSE) -> ()  [unwired: 2 in, 2 out]
        n1670 = local write "Password 2"("" ("Password")) -> ()
      }
      frame True {
        n1671 = property on="Password 2" class="Str"("Visible"=TRUE) -> ()  [unwired: 2 in, 2 out]
        n1672 = Equal?(x="Password 2", y="HFRR1234") -> (x = y?=w1780:bool)
        n1673 = case shown="True" w1780 {
          tunnel: "Password 2" -> [w1783 _]
          frame False {
            n1674 = String Length(string=w1783) -> (length=w1784:i32)
            n1675 = Greater Than 0?(x=w1784) -> (x > 0?=w1782:bool)
            n1676 = case shown="False" w1782 {
              frame False {
                n1677 = property on="Password 2" class="Str"("Caption.Text"="Password (Advance Setting)") -> ()  [unwired: 2 in, 2 out]
              }
              frame True {
                n1678 = property on="Password 2" class="Str"("Caption.Text"="Incorrect Password!") -> ()  [unwired: 2 in, 2 out]
              }
            }
          }
          frame True {
            n1679 = local write "EDIT 2"(FALSE ("EDIT 2")) -> ()
            n1680 = local write "Password 2"("" ("Password")) -> ()
            n1681 = local write "Main Tab"(T2."Advance" ("Main Tab")) -> ()
            n1682 = local write "Main Dashboard Buttons"(T1."Advance" ("Main Dashboard Buttons")) -> ()
          }
        }
      }
    }
    n1683 = case shown="True" "Prog Uno" {
      frame False {
      }
      frame True {
        n1684 = stacked-sequence {
          frame #0 {
            n1685 = Delete(path (use dialog)=path "C:/LAB-IQ-NXT/UNOCOMPILE.bat" ("working directory")) -> ()  [unwired: 4 in, 3 out]
          }
          frame #1 {
            n1686 = local read "Com Port 1"() -> (w2245:refnum<visa-resource-name>)
            n1687 = Concatenate Strings("cmd.exe /c \"mode " ("command line"), w2245, ":1200,n,8,1\"\n" ("command line")) -> (w2250:string)
            n1688 = Concatenate Strings(w2250, "CD\\\nCD WinDucom\navrdude -C avrdude.conf -v -patmega328p -carduino -P" ("command line"), w2245, " -b115200 -D -Uflash:w:UNO_V20.hex:i\n" ("command line"), "\r") -> (w2252:string)
            "STR" <- w2252
            n1689 = call <vilib>:"Write Characters To File.vi"("append to file? (new file:F)"=FALSE, "character string"=w2252, "file path (dialog if empty)"=path "C:/LAB-IQ/UNOCOMPILE.bat" ("working directory")) -> ()  [unwired: 2 in, 1 out]
          }
          frame #2 {
            n1690 = disable-structure shown="Disabled" {
              frame Disabled {
                w2256 = "cmd.exe  /c \"C:\\LAB-IQ-NXT\\UNOCOMPILE.bat\"" ("string")
                n1691 = local write "Prog Uno"(FALSE ("run minimized? (F)")) -> ()
                n1692 = call <vilib>:"System Exec.vi"("expected output size  (4096)"=u32 65535, "run minimized? (F)"=FALSE, "wait until completion? (T)"=TRUE ("run minimized? (F)"), "working directory"=path "C:/LAB-IQ-NXT", "standard input"=w2256, "command line"=w2256) -> ("error out"=w2255:errorcluster, "standard output"=→"String 42":string)  [unwired: 2 in, 2 out]
                "error out 3" <- w2255
                n1693 = flat-sequence {
                  tunnel: w2255 -> [_]
                  frame #0 {
                  }
                }
              }
              frame Enabled {
              }
            }
          }
        }
      }
    }
    n1694 = case shown="\"ISO 12156\"" "TEST STANDARD" {
      tunnel: [2.0 ("Set Temp") 0.0 ("Set Temp") 2.0 ("Set Temp") 0.0 ("Set Temp")] -> w1649
      frame "ASTM D6079", Default {
        w2202 = 50.0 ("Hz")
        w2203 = 53.0 ("Set Rh")
        w2205 = 1.0 ("Set Strk")
        w2204 = 60.0 ("Set Temp")
        # "astm hide"
        n1695 = local write "NORMAL LOAD"(200.0 ("NORMAL LOAD")) -> ()
        n1696 = local write "Set Strk"(w2205) -> ()
        n1697 = local write "Set Hz"(w2202) -> ()
        n1698 = local write "Set Temp"(w2204) -> ()
        n1699 = local write "Set Rh"(w2203) -> ()
        n1700 = local write "test time"(75.0 ("test time")) -> ()
        n1701 = local write "Set Stroke:"(w2205) -> ()
        n1702 = local write "Set Humidity:"(w2203) -> ()
        n1703 = local write "Set Frequency:"(w2202) -> ()
        n1704 = local write "Set Temperature:"(w2204) -> ()
        "Test Standard" <- "ASTM D6079" ("Test Standard 2")
      }
      frame "ISO 12156" {
        n1705 = local write "Set Strk"(1.0 ("Set Strk")) -> ()
        n1706 = local write "NORMAL LOAD"(200.0 ("NORMAL LOAD")) -> ()
        n1707 = local write "Set Temp"(60.0 ("Set Temp")) -> ()
        n1708 = local write "test time"(75.0 ("test time")) -> ()
        n1709 = local write "Set Hz"(50.0 ("Hz")) -> ()
        n1710 = local write "Set Rh"(53.0 ("Set Rh")) -> ()
      }
      frame "CEC F-096-A-06" {
        n1711 = local write "Set Strk"(1.0 ("Set Strk")) -> ()
        n1712 = local write "NORMAL LOAD"(200.0 ("NORMAL LOAD")) -> ()
        n1713 = local write "Set Temp"(60.0 ("Set Temp")) -> ()
        n1714 = local write "test time"(75.0 ("test time")) -> ()
        n1715 = local write "Set Hz"(50.0 ("Hz")) -> ()
        n1716 = local write "Set Rh"(53.0 ("Set Rh")) -> ()
      }
      frame "Custom" {
      }
    }
    n1717 = case shown="True" "Prog Due" {
      frame False {
      }
      frame True {
        n1718 = stacked-sequence {
          frame #0 {
            n1719 = Delete(path (use dialog)=path "C:/LAB-IQ/DUECOMPILE.bat" ("working directory")) -> ()  [unwired: 4 in, 3 out]
          }
          frame #1 {
            n1720 = disable-structure shown="Disabled" {
              frame Disabled {
                n1721 = local read "visa due"() -> (w2227:string)
                n1722 = Concatenate Strings("cmd.exe /c \"mode " ("command line"), w2227, ":1200,n,8,1\"\n" ("command line")) -> (w2232:string)
                n1723 = Concatenate Strings(w2232, "CD\\\nCD WinDucom\nTIMEOUT 1\n bossac.exe -i -d --port=" ("command line"), w2227, " -U false -e -w -v -b DUE.bin -R\n" ("command line"), "\r") -> (w2234:string)
                "concatenated string 2" <- w2234
                n1724 = call <vilib>:"Write Characters To File.vi"("append to file? (new file:F)"=FALSE, "character string"=w2234, "file path (dialog if empty)"=path "C:/LAB-IQ-NXT/DUECOMPILE.bat" ("working directory")) -> ()  [unwired: 2 in, 1 out]
              }
              frame Enabled {
              }
            }
          }
          frame #2 {
            # "C:\\LAB-IQ-NXT\\DUECOMPILE.bat"
            n1725 = disable-structure shown="Disabled" {
              frame Disabled {
                w2239 = "cmd.exe  /c \"C:\\LAB-IQ-NXT\\DUECOMPILE.bat\"" ("string")
                n1726 = call <vilib>:"System Exec.vi"("expected output size  (4096)"=u32 65535, "run minimized? (F)"=FALSE, "wait until completion? (T)"=TRUE ("run minimized? (F)"), "working directory"=path "C:/LAB-IQ-NXT", "standard input"=w2239, "command line"=w2239) -> ("error out"=w2238:errorcluster, "standard output"=→"String 44":string)  [unwired: 2 in, 2 out]
                "error out 4" <- w2238
                n1727 = flat-sequence {
                  tunnel: w2238 -> [_]
                  frame #0 {
                  }
                }
              }
              frame Enabled {
              }
            }
            n1728 = local write "Prog Due"(FALSE ("Prog Due")) -> ()
          }
        }
      }
    }
    n1729 = Or(x=w1646, y=w1644) -> (x .or. y?=w1645:bool)
    n1730 = case shown="\"About\"" w1643 {
      tunnel: [T25."Acquire" ("Main Tab") T25."Compare Files" ("Main Tab") T25."About" ("Main Tab")] -> w1656
      frame "Acquire", Default {
      }
      frame "Compare Files" {
      }
      frame "About" {
      }
    }
    n1731 = Or(x=w1650, y="OPEN") -> (x .or. y?=w1651:bool)
    n1732 = case shown="True" w1651 {
      tunnel: w1650 -> [_ w1791]
      frame False {
      }
      frame True {
        n1733 = stacked-sequence {
          tunnel: w1791 -> [_ w1858 _ _]
          frame #0 {
            w1807 = "  " ("String 6")
            n1734 = local write "OPEN"(FALSE ("open")) -> ()
            n1735 = local read "string1 2"() -> (w1795:string)
            n1736 = local read "string1 3"() -> (w1794:string)
            n1737 = local read "string1 4"() -> (w1793:string)
            n1738 = property on="OPEN" class="Bool (strict)"("Visible"=FALSE) -> ()  [unwired: 2 in, 2 out]
            n1739 = local write "String 6"(w1807) -> ()
            n1740 = local write "String 7"(w1807) -> ()
            n1741 = local write "String 8"(w1807) -> ()
            n1742 = local write "String 12"(w1807) -> ()
            n1743 = local read "OK Button 16"() -> (w1792:bool)
            n1744 = String To Path(string=w1795) -> (path=w1803:path)
            n1745 = String To Path(string=w1794) -> (path=w1802:path)
            n1746 = String To Path(string=w1793) -> (path=w1801:path)
            n1747 = case shown="True" w1792 {
              tunnel: [w1808 w1809] -> w1796
              frame False {
                n1748 = local read "string1"() -> (w1808:string)
              }
              frame True {
                n1749 = local read "String Indicator 4"() -> (w1809:string)
              }
            }
            n1750 = Open/Create/Replace File "Open File"(file path (use dialog)=w1803) -> (refnum out=w1799:refnum<file>)  [unwired: 5 in, 2 out]
            n1751 = Open/Create/Replace File "Open File"(file path (use dialog)=w1802) -> (refnum out=w1798:refnum<file>)  [unwired: 5 in, 2 out]
            n1752 = Open/Create/Replace File "Open File"(file path (use dialog)=w1801) -> (refnum out=w1797:refnum<file>)  [unwired: 5 in, 2 out]
            n1753 = while {
              tunnel: w1799 -> [w1821]
              i -> [w1817]
              stop <- w1816 continue-if-true
              (unwired) TRUE ("line mode (F)")
              n1754 = Read from Text File "Read File"(file (use dialog)=w1821) -> (text=w1818:string)  [unwired: 3 in, 3 out]
              n1755 = local write "Numeric 11"(w1817) -> ()
              n1756 = String Length(string=w1818) -> (length=w1820:i32)
              n1757 = Greater?(x=w1820, y=1) -> (0:w1816:bool)
            }
            n1758 = while {
              tunnel: w1798 -> [w1827]
              i -> [w1823]
              stop <- w1822 continue-if-true
              (unwired) TRUE ("line mode (F)")
              n1759 = Read from Text File "Read File"(file (use dialog)=w1827) -> (text=w1824:string)  [unwired: 3 in, 3 out]
              n1760 = local write "Numeric 12"(w1823) -> ()
              n1761 = String Length(string=w1824) -> (length=w1826:i32)
              n1762 = Greater?(x=w1826, y=1) -> (0:w1822:bool)
            }
            n1763 = while {
              tunnel: w1797 -> [w1833]
              i -> [w1829]
              stop <- w1828 continue-if-true
              (unwired) TRUE ("line mode (F)")
              n1764 = Read from Text File "Read File"(file (use dialog)=w1833) -> (text=w1830:string)  [unwired: 3 in, 3 out]
              n1765 = local write "Numeric 13"(w1829) -> ()
              n1766 = String Length(string=w1830) -> (length=w1832:i32)
              n1767 = Greater?(x=w1832, y=1) -> (0:w1828:bool)
            }
            n1768 = String To Path(string=w1796) -> (path=w1804:path)
            n1769 = Open/Create/Replace File "Open File"(file path (use dialog)=w1804) -> (refnum out=w1800:refnum<file>)  [unwired: 5 in, 2 out]
            n1770 = while {
              tunnel: w1800 -> [w1815]
              i -> [w1811]
              stop <- w1810 continue-if-true
              (unwired) TRUE ("line mode (F)")
              n1771 = Read from Text File "Read File"(file (use dialog)=w1815) -> (text=w1812:string)  [unwired: 3 in, 3 out]
              n1772 = local write "Numeric 8"(w1811) -> ()
              n1773 = String Length(string=w1812) -> (length=w1814:i32)
              n1774 = Greater?(x=w1814, y=1) -> (0:w1810:bool)
            }
          }
          frame #1 {
            w1985 = FALSE ("ACTUAL   MERGE")
            # "Sample Temp"
            # "ECR"
            # "COF"
            # "Time\nCOF\nFF\nTemp"
            n1775 = case shown="True" w1858 {
              tunnel: [w2005 w2006] -> w1859
              frame False {
                n1776 = local read "string1"() -> (w2005:string)
              }
              frame True {
                n1777 = local read "String Indicator 4"() -> (w2006:string)
              }
            }
            n1778 = local read "string1 3"() -> (w1903:string)
            n1779 = String To Path(string=w1859) -> (path=w1990:path)
            n1780 = String To Path(string=w1903) -> (path=w2001:path)
            n1781 = local read "Numeric 12"() -> (w1987:i32)
            n1782 = local read "Numeric 8"() -> (w1989:i32)
            n1783 = local read "string1 2"() -> (w1904:string)
            n1784 = local read "string1 4"() -> (w1902:string)
            n1785 = Open/Create/Replace File "Open File"(file path (use dialog)=w1990) -> (refnum out=w2004:refnum<file>, error out=w2003:errorcluster)  [unwired: 5 in, 1 out]
            n1786 = Open/Create/Replace File "Open File"(file path (use dialog)=w2001) -> (refnum out=w1997:refnum<file>, error out=w1998:errorcluster)  [unwired: 5 in, 1 out]
            n1787 = for {
              N: w1989 -> [_]
              tunnel: w2004 -> [w2152]
              tunnel: w2003 -> [w2151]
              tunnel: [w2141] -> w1916 mode=indexing
              tunnel: [w2139] -> w1973 mode=indexing
              tunnel: [w2140] -> w1968 mode=indexing
              tunnel: w1985 -> [_]
              tunnel: [w2133] -> w1970 mode=indexing
              tunnel: [w2129] -> w1939 mode=indexing
              tunnel: [w2125] -> w1914 mode=indexing
              tunnel: [w2121] -> w1895 mode=indexing
              tunnel: [w2116] -> w1855 mode=indexing
              (unwired) TRUE ("line mode (F)")
              # "freq"
              # "Stroke"
              # "Time"
              # "CoF"
              # "Humidity"
              # "Temp"
              # "Air Temp"
              # "ECR"
              n1788 = Read from Text File "Read File"(file (use dialog)=w2152, error in=w2151) -> (text=w2117:string)  [unwired: 2 in, 3 out]
              n1789 = local write "String 6"(w2117) -> ()
              n1790 = String Subset(string=w2117, offset (0)=0, length (rest)=14 ("length (rest)")) -> (substring=w2145:string)
              n1791 = String Subset(string=w2117, offset (0)=35, length (rest)=9 ("length (rest)")) -> (substring=w2142:string)
              n1792 = String Subset(string=w2117, offset (0)=15, length (rest)=9 ("length (rest)")) -> (substring=w2148:string)
              n1793 = Fract/Exp String To Number(string=w2145) -> (number=w2141:dbl)  [unwired: 3 in, 1 out]
              n1794 = Fract/Exp String To Number(string=w2142) -> (number=w2140:dbl)  [unwired: 3 in, 1 out]
              n1795 = Fract/Exp String To Number(string=w2148) -> (number=w2139:dbl)  [unwired: 3 in, 1 out]
              n1796 = String Subset(string=w2117, offset (0)=85, length (rest)=9 ("length (rest)")) -> (substring=w2118:string)
